vi "Save All.vi"(8 "error in (no error)":errorcluster, 11 "Rename in":refnum<class "ProjectItem.lvclass">) -> (0 "error out":errorcluster, 3 "Rename out":refnum<class "ProjectItem.lvclass">)   [LabVIEW 2019, in "ProjectItem.lvclass"]
uses:
  ProjectItem.lvclass
  ProjectItem.lvclass/ProjectItem.ctl
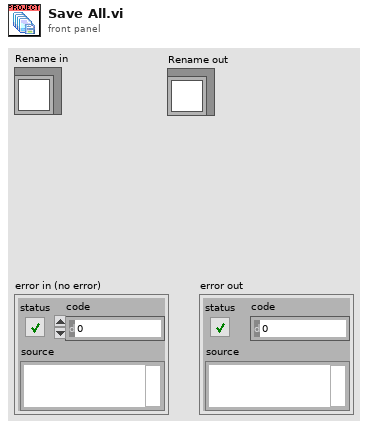
[diagram p1: front panel]
types:
  T1 = cluster{"Class":refnum<vi>, "DynamicVIs":refnum<vi>[], "StaticVIs":refnum<vi>[]}[]
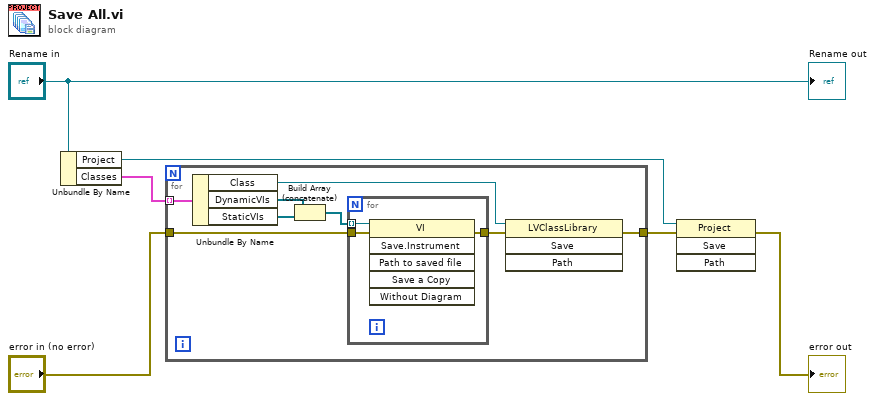
[diagram p0: block diagram]
diagram:
  n1 = Unbundle By Name("Rename in") -> ("Project"=w5:refnum<vi>, "Classes"=w1:T1)
  n2 = for {
    tunnel: w1 -> [w14] mode=indexing
    tunnel: "error in (no error)" -> [w10]
    tunnel: [w7] -> w4
    n3 = Unbundle By Name(w14) -> ("Class"=w8:refnum<vi>, "DynamicVIs"=w12:refnum<vi>[], "StaticVIs"=w13:refnum<vi>[])
    n4 = Build Array (concatenate)(w12, w13) -> (w11:refnum<vi>[])
    n5 = for {
      tunnel: w11 -> [w17] mode=indexing
      tunnel: w10 -> [w16]
      tunnel: [w15] -> w9
      n6 = invoke class="VI" method="Save.Instrument"(reference=w17, error in=w16) -> (error out=w15:errorcluster)  [unwired: 4 in, 5 out]
    }
    n7 = invoke class="LVClassLibrary" method="Save"(reference=w8, error in=w9) -> (error out=w7:errorcluster)  [unwired: 2 in, 3 out]
  }
  n8 = invoke class="Project" method="Save"(reference=w5, error in=w4) -> (error out=→"error out":errorcluster)  [unwired: 2 in, 3 out]
  "Rename out" <- "Rename in"
